vi "global_stage_initialised.vi"() -> ()   [LabVIEW 2009]
panel:
  out "Bühne initialisiert":bool
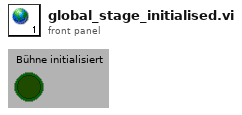
[diagram p1: front panel]
diagram:
